vi "FT Controls Change.vi"(8 "error in (no error)":errorcluster, 9 "F/T Controls Cluster Variant":variant, 11 "Rigol DG822 Square in":refnum<class "Rigol DG822 Square.lvclass">) -> (0 "error out":errorcluster, 1 "New F/T Controls Cluster Variant":variant, 3 "Rigol DG822 Square out":refnum<class "Rigol DG822 Square.lvclass">)   [LabVIEW 2021, in "Rigol DG822 UI.lvlib" / "Rigol DG822 Square.lvlib" / "Rigol DG822 Square.lvclass"]
uses:
  Rigol DG822 Square.lvclass
  Rigol DG822 UI/lib/controls.llb/FT Controls Cluster.ctl
  Rigol DG822 Square.lvclass/Rigol DG822 Square.ctl
  General/Files/lvlibp/Actors.lvlibp/Actors/Actors/Actors.lvclass
  D:/LabVIEW/General/Files/lvlibp/Actors.lvlibp/Actors/Actors/Actors.lvclass
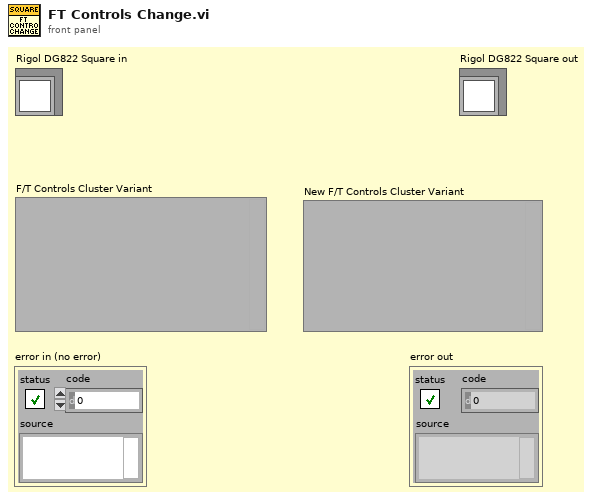
[diagram p1: front panel]
types:
  T1 = cluster{"Freq/Period":bool, "Ampl/HighL":bool, "Offset/LowL":bool}
  T2 = typedef "FT Controls Cluster.ctl" = cluster{"Freq/Period":bool, "Ampl/HighL":bool, "Offset/LowL":bool, "Duty/Width":bool}
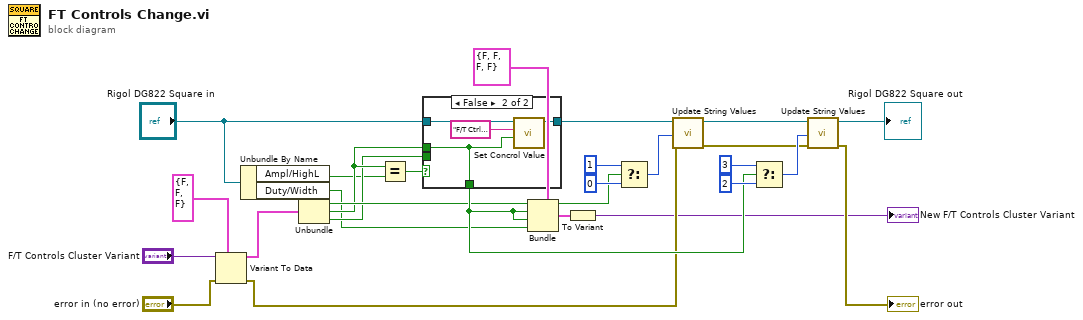
[diagram p0: block diagram]
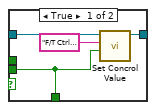
[diagram p2: hidden frame]
diagram:
  n1 = Variant To Data(error in="error in (no error)", type=T1 {"Freq/Period"=FALSE, "Ampl/HighL"=FALSE, "Offset/LowL"=FALSE} ("NewVal"), Variant="F/T Controls Cluster Variant") -> (data=w27:T1, error out=w10:errorcluster)
  n2 = Unbundle By Name("Rigol DG822 Square in") -> ("Ampl/HighL"=w3:bool, "Duty/Width"=w1:bool)
  n3 = Unbundle(w27) -> ("Freq/Period"=w11:bool, "Ampl/HighL"=w7:bool, "Offset/LowL"=w6:bool)
  n4 = Equal?(x=w7, y=w3) -> (x = y?=w12:bool)
  n5 = case shown="False" w12 {
    tunnel: [w31 w35] -> w18
    tunnel: "Rigol DG822 Square in" -> [w29 w33]
    tunnel: w6 -> [w28 _]
    tunnel: w7 -> [_ w32]
    tunnel: [w28 w32] -> w14
    frame True {
      n6 = call "Set Concrol Value.vi"("Value"=w28, "Control Label"="F/T Ctrls.Ampl/HighL", "Actors in"=w29) -> ("Actors out"=w31:refnum<class "Rigol DG822 Square.lvclass">)  [unwired: 7 in, 1 out]
    }
    frame False {
      n7 = call "Set Concrol Value.vi"("Value"=w32, "Control Label"="F/T Ctrls.Offset/LowL", "Actors in"=w33) -> ("Actors out"=w35:refnum<class "Rigol DG822 Square.lvclass">)  [unwired: 7 in, 1 out]
    }
  }
  n8 = Bundle(cluster=T2 {"Freq/Period"=FALSE, "Ampl/HighL"=FALSE, "Offset/LowL"=FALSE, "Duty/Width"=FALSE} ("F/T Ctrls"), "Freq/Period"=w11, "Ampl/HighL"=w14, "Offset/LowL"=w14, "Duty/Width"=w1) -> (w24:T2)
  n9 = To Variant(anything=w24) -> (Variant=→"New F/T Controls Cluster Variant":variant)
  n10 = Select(t=u16 1 ("Type"), s=w11, f=u16 0) -> (s? t:f=w21:u16)
  n11 = call-dynamic "Update String Values.vi"("error in (no error)"=w10, "Type"=w21, "Rigol DG822 Square in"=w18) -> ("error out"=w15:errorcluster, "Rigol DG822 Square out"=w16:refnum<class "Rigol DG822 Square.lvclass">)  [unwired: 7 in]
  n12 = Select(t=u16 3 ("Type"), s=w14, f=u16 2) -> (s? t:f=w17:u16)
  n13 = call-dynamic "Update String Values.vi"("error in (no error)"=w15, "Type"=w17, "Rigol DG822 Square in"=w16) -> ("error out"=→"error out":errorcluster, "Rigol DG822 Square out"=→"Rigol DG822 Square out":refnum<class "Rigol DG822 Square.lvclass">)  [unwired: 7 in]
